vi "comet_try_open.vi"(7 "idn":bool, 8 "error in":errorcluster, 11 "thermo in":T1={"type"=enum."COMET Tx5xx (ethernet)", "comment"="", "tag"="", "refresh"=0.0, "IP"="", "port"=0, "VISA"="", "last readout"=timestamp(0 s since 1904-01-01), "TCP ref"=refnum, "VISA sess"="", "idn"="", "press"=0.0, "RH"=0.0, "temp"=0.0, "pres cor"=[], "RH cor"=[], "temp cor"=[], "try left"=0, "failed"=FALSE, "RTD set"=[], "RTD inv"=[], "range"=0.0, "net mode"=enum."MODBUS", "try fail"=enum."Stop trying - return NaN", "timeout [s]"=0.0, "max retries"=0, "sim t [deg]"=0.0} {"RTD inv" format="%.1f"; "RTD set" format="%.1f"; "temp cor" format="%.1f"; "RH cor" format="%.1f"; "pres cor" format="%.1f"; "refresh" min=0.1 max=1000.0 format="%.2f"}) -> (0 "error out":errorcluster, 3 "thermo cluster":T1={"type"=enum."COMET Tx5xx (ethernet)", "comment"="", "tag"="", "refresh"=5.0, "IP"="", "port"=502, "VISA"="", "last readout"=timestamp(0 s since 1904-01-01), "TCP ref"=refnum, "VISA sess"="", "idn"="", "press"=0.0, "RH"=0.0, "temp"=0.0, "pres cor"=[], "RH cor"=[], "temp cor"=[], "try left"=0, "failed"=FALSE, "RTD set"=[], "RTD inv"=[], "range"=0.0, "net mode"=enum."MODBUS", "try fail"=enum."Stop trying - return NaN", "timeout [s]"=0.0, "max retries"=0, "sim t [deg]"=0.0} {"RTD inv" format="%.1f"; "RTD set" format="%.1f"; "temp cor" format="%.1f"; "RH cor" format="%.1f"; "pres cor" format="%.1f"; "refresh" min=0.1 max=1000.0 format="%.2f"}, 4 "name":string)   [LabVIEW 2020]
uses:
  thermo.ctl
  thermo_types.ctl
  Thermometer Fail Action.ctl
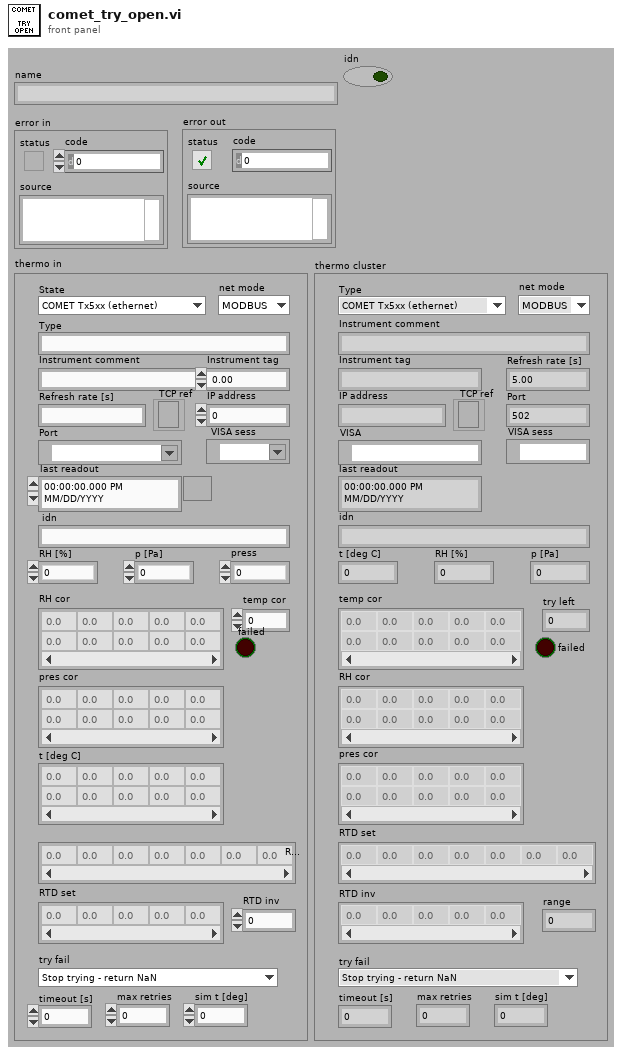
[diagram p1: front panel]
types:
  T1 = typedef "thermo.ctl" = cluster{"type":T2, "comment":string, "tag":string, "refresh":dbl, "IP":string, "port":u16, "VISA":refnum<visa-resource-name>, "last readout":timestamp, "TCP ref":refnum<k5>, "VISA sess":refnum<visa-resource-name>, "idn":string, "press":dbl, "RH":dbl, "temp":dbl, "pres cor":dbl[][], "RH cor":dbl[][], "temp cor":dbl[][], "try left":i32, "failed":bool, "RTD set":dbl[], "RTD inv":dbl[], "range":dbl, "net mode":enum16{"MODBUS", "HTTP"}, "try fail":T3, "timeout [s]":dbl, "max retries":i32, "sim t [deg]":dbl}
  T2 = typedef "thermo_types.ctl" = enum16{"Disabled", "Simulated", "COMET Tx5xx (ethernet)", "Keithley 2002 (GPIB) + RTD", "Agilent 344xx (GPIB) + RTD"}
  T3 = typedef "Thermometer Fail Action.ctl" = enum16{"Stop trying - keep last value", "Stop trying - return NaN", "Generate error - stop sweep"}
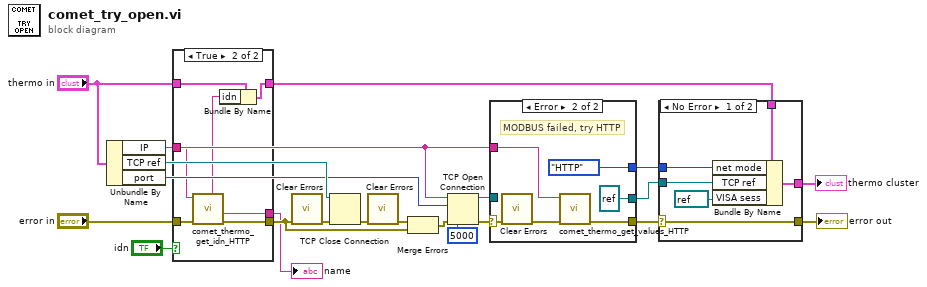
[diagram p0: block diagram]
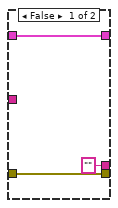
[diagram p2: hidden frame]
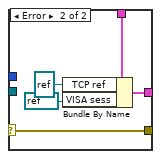
[diagram p3: hidden frame]
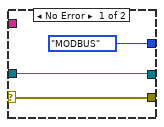
[diagram p4: hidden frame]
diagram:
  n1 = Unbundle By Name("thermo in") -> ("IP"=w11:string, "TCP ref"=w15:refnum<k5>, "port"=w14:u16)
  n2 = case shown="True" "idn" {
    tunnel: [w23 w31] -> w16
    tunnel: ["" ("name") w30] -> w13
    tunnel: w11 -> [_ w29]
    tunnel: "error in" -> [w23 w28]
    tunnel: "thermo in" -> [w22 w27]
    tunnel: [w22 w26] -> w1
    frame False {
    }
    frame True {
      n3 = call "comet_thermo_get_idn_HTTP.vi"("error in"=w28, "IP"=w29) -> ("error out"=w31:errorcluster, "name"=w30:string, "ID string (virtual)"=w25:string)  [unwired: 3 in, 4 out]
      n4 = Bundle By Name(cluster=w27, "idn"=w25) -> (w26:T1)
    }
  }
  "name" <- w13
  n5 = call <vilib>:"Clear Errors.vi"("error in (no error)"=w16) -> ("error out"=w19:errorcluster)  [unwired: 5 in, 1 out]
  n6 = TCP Close Connection(connection ID=w15, error in (no error)=w19) -> (error out=w20:errorcluster)  [unwired: 1 in, 1 out]
  n7 = call <vilib>:"Clear Errors.vi"("error in (no error)"=w20) -> ("error out"=w18:errorcluster)  [unwired: 5 in, 1 out]
  n8 = Merge Errors(w18, w16) -> (w17:errorcluster)
  n9 = TCP Open Connection(address=w11, remote port or service name=w14, timeout ms (60000)=5000, error in (no error)=w17) -> (connection ID=w8:refnum<k5>, error out=w12:errorcluster)  [unwired: 1 in]
  n10 = case shown="Error" w12 {
    selector: w12 -> [w34 w36]
    tunnel: w11 -> [_ w40]
    tunnel: [w34 w39] -> w5
    tunnel: [enum16{"MODBUS", "HTTP"}."MODBUS" ("net mode") enum16{"MODBUS", "HTTP"}."HTTP" ("net mode")] -> w9
    tunnel: [w32 refnum<k5> refnum ("connection ID")] -> w7
    tunnel: w8 -> [w32 _]
    frame No Error {
    }
    frame Error {
      # "MODBUS failed, try HTTP"
      n11 = call <vilib>:"Clear Errors.vi"("error in (no error)"=w36) -> ("error out"=w35:errorcluster)  [unwired: 5 in, 1 out]
      n12 = call "comet_thermo_get_values_HTTP.vi"("error in"=w35, "IP"=w40) -> ("error out"=w39:errorcluster)  [unwired: 5 in, 4 out]
    }
  }
  n13 = case shown="No Error" w5 {
    selector: w5 -> [w41 w48]
    tunnel: w1 -> [w46 w51]
    tunnel: w9 -> [w45 _]
    tunnel: w7 -> [w44 _]
    tunnel: [w42 w49] -> w6
    tunnel: [w41 w48] -> w4
    frame No Error {
      n14 = Bundle By Name(cluster=w46, "net mode"=w45, "TCP ref"=w44, "VISA sess"=refnum<visa-resource-name> refnum) -> (w42:T1)
    }
    frame Error {
      n15 = Bundle By Name(cluster=w51, "TCP ref"=refnum<k5> refnum, "VISA sess"=refnum<visa-resource-name> refnum) -> (w49:T1)
    }
  }
  "thermo cluster" <- w6
  "error out" <- w4
